vi "RT Driver VI.vi"(7 "Operation":T1, 11 "Device Reference in":T2 format="%.0x") -> (0 "Error Code":i32)   [LabVIEW 2019, in "Diagnostics Addon Engine.lvlib"]
uses:
  Diagnostics Addon Engine.lvlib
  <vilib>/NI VeriStand/Custom Device API/Custom Device Item Ref.ctl
  <vilib>/NI VeriStand/Custom Device API/Hardware Interface Driver VI Operation.ctl
  <vilib>/NI/NIVS Inline Async API/_VS Inline Async API/VS Inline Async API/VS Inline Async API.lvclass
  Addon Shared/Types/SysDef.Compile.ctl
  Addon Shared/Types/CAN.ctl
  Addon Shared/Types/CAN.Interface.ctl
  Addon Shared/Types/Protocol.ctl
  Addon Shared/Types/Transport.ctl
  Addon Shared/Types/986x.ctl
  Addon Shared/Types/Frame.Compile.ctl
  Addon Shared/Types/Type.ctl
  Addon Shared/Types/Signal.ctl
  Addon Shared/Types/DPID.ctl
  Addon Shared/Types/DPID.Rate.ctl
  Addon Shared/Types/DTC.Settings.ctl
  Addon Shared/Types/DTC.Descriptor.ctl
  Addon Shared/Types/Poll.Compiled.ctl
  Addon Shared/Types/Security.ctl
  Addon Shared/Types/Security.Type.ctl
  <vilib>/NI/NIVS Inline Async API/_VS Inline Async API/VS Inline Async API/Types/Error Handling Settings.ctl
  <vilib>/NI/NIVS Inline Async API/_VS Inline Async API/VS Inline Async API/VS Inline Async API.lvclass/VS Inline Async API.ctl
  <vilib>/NI/NIVS Inline Async API/_Data Access Engine/Data Access Engine/Data Access Engine.lvclass/Data Access Engine.ctl
  <vilib>/NI/NIVS Inline Async API/_Data Access Engine/Access Type Classes/Write/Write.lvclass/Write.ctl
  <vilib>/NI/NIVS Inline Async API/_Data Access Engine/Access Type Classes/ReadWrite/ReadWrite.lvclass/ReadWrite.ctl
  <vilib>/NI/NIVS Inline Async API/_Data Access Engine/Access Type Classes/Read/Read.lvclass/Read.ctl
  <vilib>/NI/NIVS Inline Async API/_Data Access Engine/Data Access Engine/Methods/Data.Engine.Read Data from HW.vi
  <vilib>/NI/NIVS Inline Async API/_VS Inline Async API/Error Handling Process/SubVIs/Error.GetError.vi
  <vilib>/NI/NIVS Inline Async API/_Data Access Engine/Data Access Engine/Methods/Data.Engine.Write Data to HW.vi
  <vilib>/NI/NIVS Inline Async API/_Data Access Engine/Access Type Classes/ReadWrite/ReadWrite.EngineData.vi
  <vilib>/NI/NIVS Inline Async API/_Data Access Engine/Access Type Classes/Write/Write.EngineData.vi
  <vilib>/NI/NIVS Inline Async API/_Data Access Engine/Access Type Classes/Read/Read.EngineData.vi
  <vilib>/NI VeriStand/Custom Device API/NI VeriStand - Get Channel Value by Data Reference.vi
  <vilib>/NI VeriStand/Custom Device API/NI VeriStand - Set Channel Value by Data Reference.vi
  <vilib>/NI VeriStand/Custom Device API/NI VeriStand - Get Channel Values by Block Data Reference.vi
  Addon Shared/SubVIs/Constants.vi
  <vilib>/NI VeriStand/Custom Device API/Get Item Property (Variant).vi
  <vilib>/Utility/SystemLogging/Write to System Log.vi
  SubVIs/Bitfile.Initialize.vi
  <vilib>/NI VeriStand/Custom Device API/Global Data Refs.vi
  Addon Shared/Diagnostics Addon Shared.lvlib
  <vilib>/NI VeriStand/Custom Device API/Custom Device API.lvlib
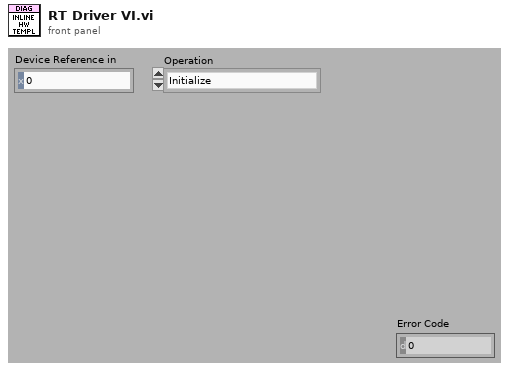
[diagram p1: front panel]
types:
  T1 = typedef "Custom Device API.lvlib/Hardware Interface Driver VI Operation.ctl" = enum16{"Initialize", "Start", "Read Data from HW", "Write Data to HW", "Close"}
  T2 = typedef "Custom Device API.lvlib/Custom Device Item Ref.ctl" = u64
  T3 = cluster{"Device Error":errorcluster, "FPGA Session":u32, "Async":refnum<class "VS Inline Async API.lvclass">}
  T4 = typedef "Diagnostics Addon Shared.lvlib/SysDef.Compile.ctl" = cluster{"Name":string, "CAN":T5, "986x":T9, "Reads":T10[], "Frames Lookup":variant, "Writes":T10[], "DPIDs":T13[], "DPID Lookup":variant, "DTC":T15, "Created DTCs":u32, "Polls":T17[], "Service Channels Status Lookup":variant, "Trigger Lookup":variant, "Security":T18}
  T5 = typedef "Diagnostics Addon Shared.lvlib/CAN.ctl" = cluster{"Interface":T6, "Baud Rate":u64, "Diagnostic Protocol":T7, "Transport Protocol":T8, "Transmit ID":u32, "Receive ID":u32, "Transmit Extension":u8, "Receive Extension":u8, "Receive UUDT ID":u32, "Enable Stream":bool, "VW TP Channel ID":u32, "Fill Frame":bool, "Fill Byte":u8, "Termination":bool, "LIN Cluster":refnum<k21>, "NAD":u8, "IO Mode":u32, "Max DLC":u16, "FD Baud Rate":u64, "Timeout":u32}
  T6 = typedef "Diagnostics Addon Shared.lvlib/CAN.Interface.ctl" = string
  T7 = typedef "Diagnostics Addon Shared.lvlib/Protocol.ctl" = enum16{"GMLAN", "KWP-2000", "UDS", "User-Defined"}
  T8 = typedef "Diagnostics Addon Shared.lvlib/Transport.ctl" = enum16{"ISO TP - Normal Mode", "ISO TP - Mixed Mode", "VW TP 2.0", "Diagnostics on IP", "ISO TP LIN"}
  T9 = typedef "Diagnostics Addon Shared.lvlib/986x.ctl" = cluster{"Enable":bool, "RIO Device":string, "Bitfile":path}
  T10 = typedef "Diagnostics Addon Shared.lvlib/Frame.Compile.ctl" = cluster{"ID":u32, "Type":T11, "Signals":T12[]}
  T11 = typedef "Diagnostics Addon Shared.lvlib/Type.ctl" = enum16{"DID", "CDID", "PID", "CPID", "Read Memory", "Write Memory", "IO Control", "Routine Start", "Routine Request", "Routine Stop", "User Defined", "DTC Control", "Clear DTCs", "Read DTCs", "Start DTCs", "DTC Change Count", "Tester Present", "Unlock ECU", "Reset ECU", "Diag Session Control", "Communication Control", "DPID Control", "Poll Control", "Diag CAN Control"}
  T12 = typedef "Diagnostics Addon Shared.lvlib/Signal.ctl" = cluster{"Start Bit":u32, "Length":u32, "Scaling Factor":dbl, "Scaling Offset":dbl, "Minimum":dbl, "Maximum":dbl, "Data Type":u32, "Byte Order":u32, "Default Value":dbl, "Name":string, "Units":string}
  T13 = typedef "Diagnostics Addon Shared.lvlib/DPID.ctl" = cluster{"DPID ID":u8, "Speed":T14, "PIDs":u16[]}
  T14 = typedef "Diagnostics Addon Shared.lvlib/DPID.Rate.ctl" = enum16{"Slow", "Medium", "Fast"}
  T15 = typedef "Diagnostics Addon Shared.lvlib/DTC.Settings.ctl" = cluster{"Descriptor":T16, "Value.Code":dbl[], "Value.String":string[], "Value.J2012String":string[], "Status.Code":dbl[], "Status.String":string[]}
  T16 = typedef "Diagnostics Addon Shared.lvlib/DTC.Descriptor.ctl" = cluster{"DTC Byte Length":i32, "Status Byte Length":i32, "Add Data Byte Length":i32, "Byte Order":enum16{"Motorola", "Intel"}}
  T17 = typedef "Diagnostics Addon Shared.lvlib/Poll.Compiled.ctl" = cluster{"Speed":T14, "DID IDs":u32[], "PID IDs":u32[]}
  T18 = typedef "Diagnostics Addon Shared.lvlib/Security.ctl" = cluster{"Type":T19, "Source DLL Path":path, "Target DLL Path":path, "Security Level":u8}
  T19 = typedef "Diagnostics Addon Shared.lvlib/Security.Type.ctl" = enum16{"None", "DLL", "MasterKey"}
  T20 = cluster{"FPGA Session":u32, "Async":refnum<class "VS Inline Async API.lvclass">, "VS References":T4}
  T21 = typedef "VS Inline Async API.lvlib/VS Inline Async API.lvclass/Error Handling Settings.ctl" = cluster{"Write to SystemLog (F)":bool}
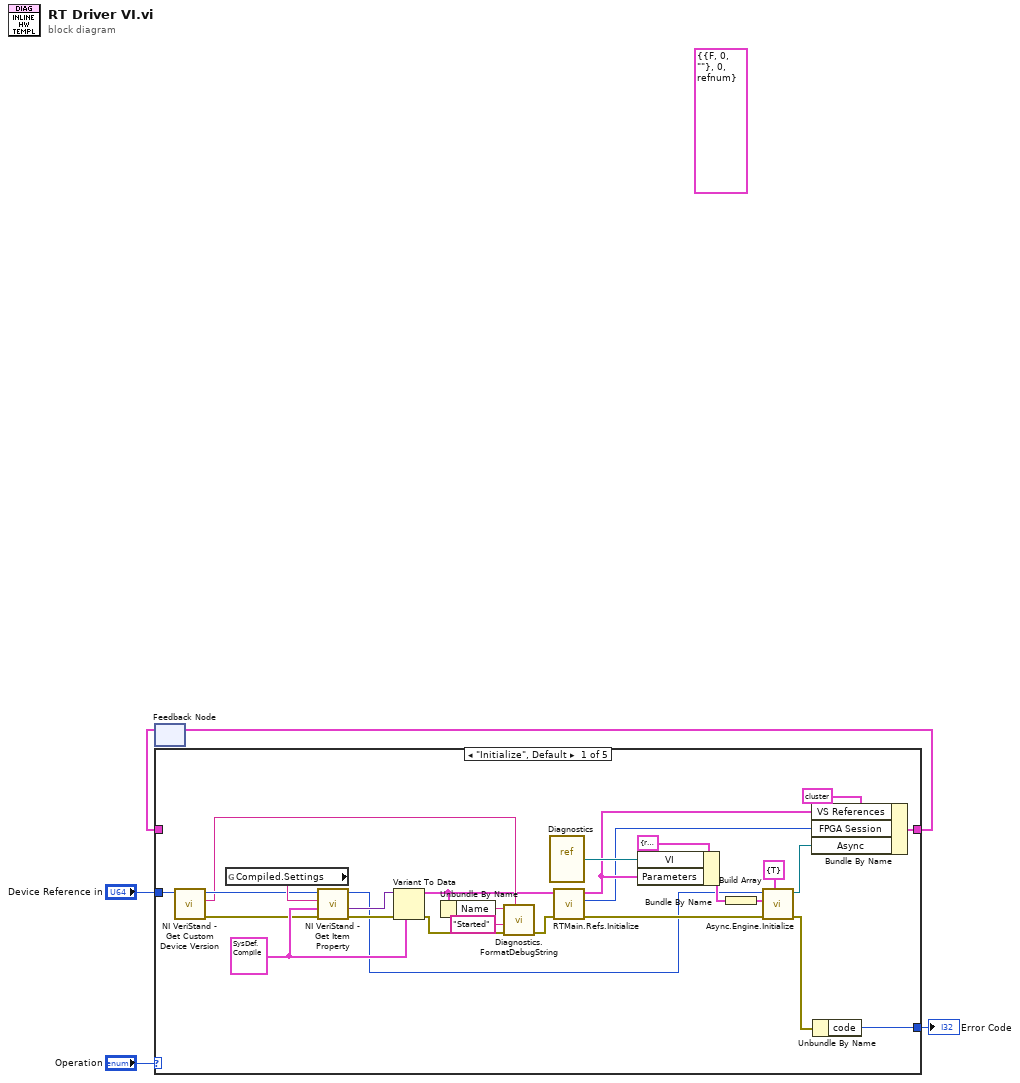
[diagram p0: block diagram]
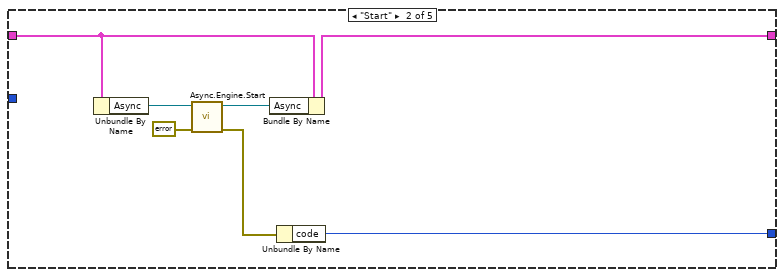
[diagram p2: hidden frame]
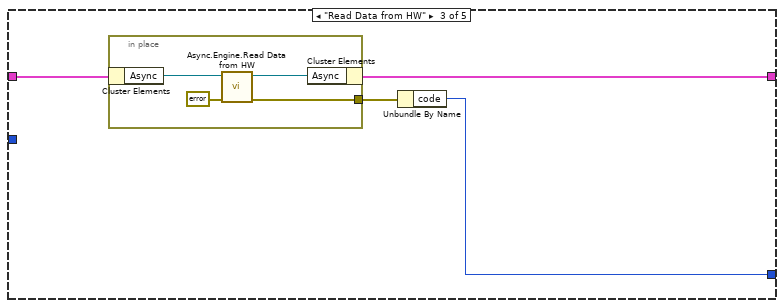
[diagram p3: hidden frame]
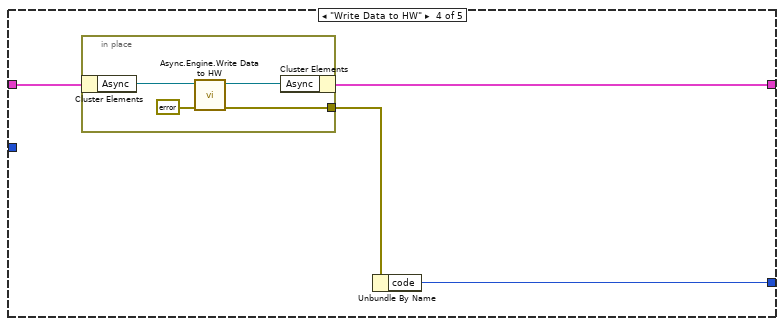
[diagram p4: hidden frame]
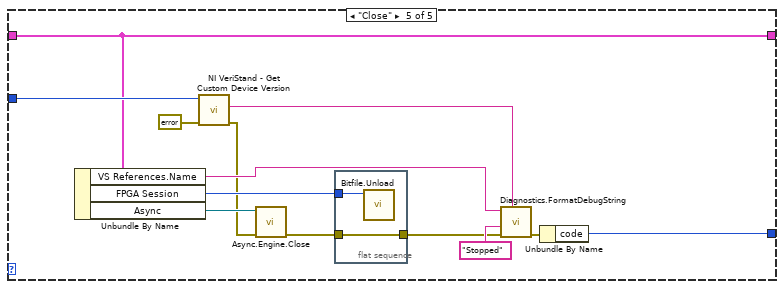
[diagram p5: hidden frame]
diagram:
  (unwired) T3 {"Device Error"={"status"=FALSE, "code"=0, "source"=""}, "FPGA Session"=0, "Async"=refnum} ("cluster")
  n1 = feedback #1() -> (w3:T20)  [unwired: 1 out]
  n2 = case shown="\"Initialize\", Default" "Operation" {
    tunnel: [w32 w38 w42 w50 w58] -> w2
    tunnel: w3 -> [_ w39 w43 w51 w58]
    tunnel: "Device Reference in" -> [w19 _ _ _ w65]
    tunnel: [w6 w34 w40 w48 w59] -> w1
    frame "Initialize", Default {
      w28 = T4 {"Name"="", "CAN"={"Interface"="", "Baud Rate"=0, "Diagnostic Protocol"=enum."GMLAN", "Transport Protocol"=enum."ISO TP - Normal Mode", "Transmit ID"=0, "Receive ID"=0, "Transmit Extension"=0, "Receive Extension"=0, "Receive UUDT ID"=0, "Enable Stream"=FALSE, "VW TP Channel ID"=0, "Fill Frame"=FALSE, "Fill Byte"=0, "Termination"=FALSE, "LIN Cluster"="", "NAD"=0, "IO Mode"=0, "Max DLC"=0, "FD Baud Rate"=0, "Timeout"=0}, "986x"={"Enable"=FALSE, "RIO Device"="", "Bitfile"=path ""}, "Reads"=[], "Frames Lookup"=variant, "Writes"=[], "DPIDs"=[], "DPID Lookup"=variant, "DTC"={"Descriptor"={"DTC Byte Length"=0, "Status Byte Length"=1, "Add Data Byte Length"=1, "Byte Order"=enum."Motorola"}, "Value.Code"=[], "Value.String"=[], "Value.J2012String"=[], "Status.Code"=[], "Status.String"=[]}, "Created DTCs"=0, "Polls"=[], "Service Channels Status Lookup"=variant, "Trigger Lookup"=variant, "Security"={"Type"=enum."None", "Source DLL Path"=path "", "Target DLL Path"=path "", "Security Level"=0}} ("VS References")
      n3 = call <vilib>:"NI VeriStand - Get Custom Device Version.vi"("Device Ref in"=w19) -> ("error out"=w17:errorcluster, "Value"=w16:string, "Device Ref out"=w18:T2)  [unwired: 8 in]
      n4 = global read "Constants.vi" "Compiled.Settings"() -> (w31:string)
      n5 = call-poly <vilib>:"NI VeriStand - Get Item Property.vi"("error in (no error)"=w17, "Default Value"=w28, "Property Name"=w31, "Item Ref in"=w18) -> ("error out"=w30:errorcluster, "Value"=w29:variant, "Item Ref out"=w22:T2)  [unwired: 4 in, 1 out]
      n6 = Variant To Data(error in=w30, type=w28, Variant=w29) -> (data=w10:T4, error out=w12:errorcluster)
      n7 = Unbundle By Name(w10) -> ("Name"=w15:string)
      n8 = call "Diagnostics.FormatDebugString.vi"("Version"=w16, "error in (no error)"=w12, "State"="Started" ("string"), "Name"=w15) -> ("error out"=w11:errorcluster)  [unwired: 7 in]
      n9 = vi-ref "Diagnostics.vi"() -> (w26:refnum<vi>)
      n10 = call "RTMain.Refs.Initialize.vi"("error in (no error)"=w11, "VS References"=w10) -> ("error out"=w23:errorcluster, "FPGA Session"=w7:u32, "VS Main Configuration"=w9:T4)  [unwired: 7 in]
      n11 = Bundle By Name(cluster=cluster{"VI":refnum<vi>, "Parameters":variant} {"VI"=refnum, "Parameters"=variant} ("Process"), "VI"=w26, "Parameters"=w9) -> (w25:cluster{"VI":refnum<vi>, "Parameters":variant})
      n12 = Build Array(w25) -> (w24:cluster{"VI":refnum<vi>, "Parameters":variant}[])
      n13 = call <vilib>:"Async.Engine.Initialize.vi"("Error Log Settings"=T21 {"Write to SystemLog (F)"=TRUE}, "error in (no error)"=w23, "Processes"=w24, "Custom Device Ref"=w22) -> ("error out"=w21:errorcluster, "Async"=w20:refnum<class "VS Inline Async API.lvclass">)  [unwired: 6 in]
      n14 = Bundle By Name(cluster=T20 {"FPGA Session"=0, "Async"=refnum, "VS References"={"Name"="", "CAN"={"Interface"="", "Baud Rate"=0, "Diagnostic Protocol"=enum."GMLAN", "Transport Protocol"=enum."ISO TP - Normal Mode", "Transmit ID"=0, "Receive ID"=0, "Transmit Extension"=0, "Receive Extension"=0, "Receive UUDT ID"=0, "Enable Stream"=FALSE, "VW TP Channel ID"=0, "Fill Frame"=FALSE, "Fill Byte"=0, "Termination"=FALSE, "LIN Cluster"="", "NAD"=0, "IO Mode"=0, "Max DLC"=0, "FD Baud Rate"=0, "Timeout"=0}, "986x"={"Enable"=FALSE, "RIO Device"="", "Bitfile"=path ""}, "Reads"=[], "Frames Lookup"=variant, "Writes"=[], "DPIDs"=[], "DPID Lookup"=variant, "DTC"={"Descriptor"={"DTC Byte Length"=0, "Status Byte Length"=1, "Add Data Byte Length"=1, "Byte Order"=enum."Motorola"}, "Value.Code"=[], "Value.String"=[], "Value.J2012String"=[], "Status.Code"=[], "Status.String"=[]}, "Created DTCs"=0, "Polls"=[], "Service Channels Status Lookup"=variant, "Trigger Lookup"=variant, "Security"={"Type"=enum."None", "Source DLL Path"=path "", "Target DLL Path"=path "", "Security Level"=0}}}, "VS References"=w9, "FPGA Session"=w7, "Async"=w20) -> (w32:T20)
      n15 = Unbundle By Name(w21) -> ("code"=w6:i32)
    }
    frame "Start" {
      n16 = Unbundle By Name(w39) -> ("Async"=w36:refnum<class "VS Inline Async API.lvclass">)
      n17 = call <vilib>:"Async.Engine.Start.vi"("error in (no error)"=errorcluster {"status"=FALSE, "code"=0, "source"=""} ("error out"), "VS Inline Async API in"=w36) -> ("error out"=w37:errorcluster, "VS Inline Async API out"=w35:refnum<class "VS Inline Async API.lvclass">)  [unwired: 8 in]
      n18 = Bundle By Name(cluster=w39, "Async"=w35) -> (w38:T20)
      n19 = Unbundle By Name(w37) -> ("code"=w34:i32)
    }
    frame "Read Data from HW" {
      n20 = in-place {
        in-place-border: [w45] -> w41
        n21 = in-place-cluster #2(w43) -> ("Async"=w47:refnum<class "VS Inline Async API.lvclass">)
        n22 = call <vilib>:"Async.Engine.Read Data from HW.vi"("error in"=errorcluster {"status"=FALSE, "code"=0, "source"=""} ("error out"), "Async in"=w47) -> ("error out"=w45:errorcluster, "Async out"=w46:refnum<class "VS Inline Async API.lvclass">)  [unwired: 8 in]
        n23 = in-place-cluster #2("Async"=w46) -> (w42:T20)
      }
      n24 = Unbundle By Name(w41) -> ("code"=w40:i32)
    }
    frame "Write Data to HW" {
      n25 = in-place {
        in-place-border: [w53] -> w49
        n26 = in-place-cluster #3(w51) -> ("Async"=w55:refnum<class "VS Inline Async API.lvclass">)
        n27 = call <vilib>:"Async.Engine.Write Data to HW.vi"("error in (no error)"=errorcluster {"status"=FALSE, "code"=0, "source"=""} ("error out"), "VS Inline Async API in"=w55) -> ("error out"=w53:errorcluster, "VS Inline Async API out"=w54:refnum<class "VS Inline Async API.lvclass">)  [unwired: 8 in]
        n28 = in-place-cluster #3("Async"=w54) -> (w50:T20)
      }
      n29 = Unbundle By Name(w49) -> ("code"=w48:i32)
    }
    frame "Close" {
      n30 = Unbundle By Name(w58) -> ("VS References.Name"=w60:string, "FPGA Session"=w68:u32, "Async"=w67:refnum<class "VS Inline Async API.lvclass">)
      n31 = call <vilib>:"NI VeriStand - Get Custom Device Version.vi"("error in (no error)"=errorcluster {"status"=FALSE, "code"=0, "source"=""} ("error out"), "Device Ref in"=w65) -> ("error out"=w56:errorcluster, "Value"=w63:string)  [unwired: 7 in, 1 out]
      n32 = call <vilib>:"Async.Engine.Close.vi"("error in (no error)"=w56, "Async in"=w67) -> ("error out"=w66:errorcluster)  [unwired: 8 in, 1 out]
      n33 = flat-sequence {
        tunnel: [w69] -> w61
        tunnel: w66 -> [w69]
        tunnel: w68 -> [w70]
        frame #0 {
          n34 = call "Bitfile.Unload.vi"("Session"=w70) -> ()  [unwired: 11 in]
        }
      }
      n35 = call "Diagnostics.FormatDebugString.vi"("Version"=w63, "error in (no error)"=w61, "State"="Stopped" ("string"), "Name"=w60) -> ("error out"=w62:errorcluster)  [unwired: 7 in]
      n36 = Unbundle By Name(w62) -> ("code"=w59:i32)
    }
  }
  "Error Code" <- w1
  n37 = feedback-in #1(w2) -> ()
